vi "Obtain Message Transport.vi"(11 "Message Transport":refnum<class "Message Transport.lvclass">) -> (0 "error out":errorcluster, 3 "Message Transport out":refnum<class "Message Transport.lvclass">)   [LabVIEW 2018, in "Message Transport.lvclass"]
uses:
  Message Transport.lvclass
  Message_class/Message.lvclass
  Message Transport.lvclass/Message Transport.ctl
  Communication_class/Set Message Queue.vi
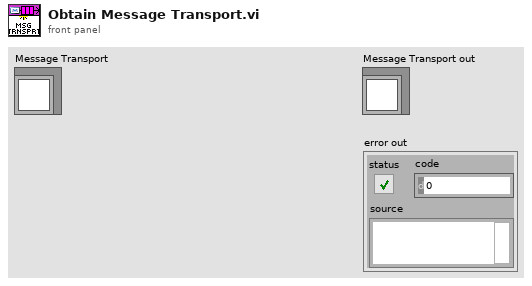
[diagram p1: front panel]
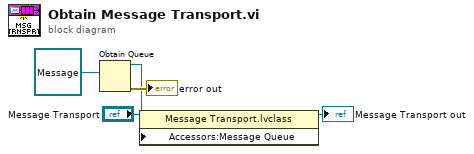
[diagram p0: block diagram]
diagram:
  n1 = Obtain Queue(element data type=refnum<class "Message.lvclass"> refnum ("Message in")) -> (queue out=w2:refnum<queue>, error out=→"error out":errorcluster)  [unwired: 4 in, 1 out]
  n2 = property class="Message Transport.lvclass"(reference="Message Transport", "Accessors:Message Queue"=w2) -> (reference out=→"Message Transport out":refnum<class "Message Transport.lvclass">)  [unwired: 1 in, 1 out]
